vi "Connection Engine.vi"(8 "error in (no error)":errorcluster, 11 "State Variables":T1={"TCP Refs"={"Connection List"=refnum, "listener ID"=refnum}, "Stop"=refnum, "Top VI"=refnum, "Parameters"={"Properties"={"Name"="", "CAN"={"Database File"=path "", "CAN Interface"=enum."CAN0", "Baud Rate"=0, "Diagnostic Protocol"=enum."GMLAN", "Transport Protocol"=enum."ISO TP - Normal Mode", "Transmit ID"=0, "Receive ID"=0, "Transmit Extension"=0, "Receive Extension"=0, "Receive UUDT ID"=0, "Enable Stream"=TRUE, "VW TP Channel ID"=0, "Security"={"DLL Path"=path "", "Security Level"=1}}, "FPGA Settings"={"RT Bitfile Path"=path "", "RIO Device"=0, "Enable"=FALSE}, "PIDs"=[], "PID Lookup"=variant, "CPIDs"=[], "CPID Lookup"=variant, "DIDs"=[], "DID Lookup"=variant, "DPIDs"=[], "DPID Lookup"=variant, "DTC descriptor"={"DTC Byte Length"=2, "Status Byte Length"=1, "Add Data Byte Length"=1, "Byte Order"=enum."Motorola"}}, "ChanRefs"={"ToVS.PIDs"={"Name"="", "Write to VS Engine FIFO"=refnum, "Pairs"={"Refs"=[], "Values"=[]}}, "ToVS.DIDs"={"Name"="", "Write to VS Engine FIFO"=refnum, "Pairs"={"Refs"=[], "Values"=[]}}, "ToVS.DTCs"={"Name"="", "Write to VS Engine FIFO"=refnum, "Pairs"={"Refs"=[], "Values"=[]}}, "ToVS.DTCCount"={"Name"="", "Write to VS Engine FIFO"=refnum, "Pairs"={"Refs"=[], "Values"=[]}}, "ToVS.Success"={"Name"="", "Write to VS Engine FIFO"=refnum, "Pairs"={"Refs"=[], "Values"=[]}}, "FromVS.CPIDs"={"Name"="", "Read from VS Engine FIFO"=refnum, "Pairs"={"Refs"=[], "Values"=[]}}, "Cmds"={"Name"="", "Write to VS Engine FIFO"=refnum, "Read from VS Engine FIFO"=refnum, "Pairs"={"Chan Refs"=[], "Prev. Values"=[]}}}}, "ADCS Connection"={"Diag CAN Handle"=0, "Transport Protocol"=enum."ISO TP - Normal Mode", "Receive Address Extension"=0, "Transmit Address Extension"=0, "Receive CAN Id"=0, "Transmit CAN Id"=0, "Diag CAN Queue"=refnum, "Log Frames ?"=FALSE, "My TP Address"=0, "Other TP Address"=0, "T1"=0, "T2"=0, "T3"=0, "T4"=0, "Tx SN"=0, "Block Size"=0, "Rx SN"=0, "VW TP Initialized?"=FALSE, "Tx block no"=0, "baud rate"=0, "Interface"="", "Channel Diag CAN Handle"=0, "UDP Connection ID"=refnum, "TCP Connection ID"=refnum, "Target IP Addr"=0, "Source Address"=0, "Target Address"=0, "Send Header NACK?"=FALSE, "DLL Handle"=0, "NAD"=0, "Time Stamp read first"=0.0, "Time Stamp read last"=0.0, "Time Stamp write first"=0.0, "Time Stamp write last"=0.0, "Time Stamp write"=0.0, "Time Stamp read"=0.0}, "XNET References"={"Database"="", "GMLAN DPID Session"="", "Cluster"=""}, "BufferedCmds"=refnum, "XNETEngine (GMLAN)"=refnum} {"Parameters"."ChanRefs"."Cmds"."Pairs"."Chan Refs" format="%.0x"; "Parameters"."ChanRefs"."ToVS.Success"."Pairs"."Refs" format="%.0x"; "Parameters"."ChanRefs"."ToVS.DTCCount"."Pairs"."Refs" format="%.0x"; "Parameters"."ChanRefs"."ToVS.DTCs"."Pairs"."Refs" format="%.0x"; "Parameters"."ChanRefs"."ToVS.PIDs"."Pairs"."Refs" format="%.0x"; "Parameters"."ChanRefs"."ToVS.DIDs"."Pairs"."Refs" format="%.0x"; "Parameters"."Properties"."CPIDs"."Signals"."Byte Order" items=["Little Endian", "Big Endian"]; "Parameters"."Properties"."CPIDs"."Signals"."Data Type" items=["Signed", "Unsigned", "IEEE Float"]; "Parameters"."Properties"."DIDs"."Signals"."Byte Order" items=["Little Endian", "Big Endian"]; "Parameters"."Properties"."DIDs"."Signals"."Data Type" items=["Signed", "Unsigned", "IEEE Float"]; "Parameters"."Properties"."CAN"."VW TP Channel ID" format="%.0x"; "Parameters"."Properties"."CAN"."Receive UUDT ID" format="%.0x"; "Parameters"."Properties"."CAN"."Receive Extension" format="%.0x"; "Parameters"."Properties"."CAN"."Transmit Extension" format="%.0x"; "Parameters"."Properties"."CAN"."Receive ID" format="%.0x"; "Parameters"."Properties"."CAN"."Transmit ID" format="%.0x"; "Parameters"."Properties"."PIDs"."Signals"."Byte Order" items=["Little Endian", "Big Endian"]; "Parameters"."Properties"."PIDs"."Signals"."Data Type" items=["Signed", "Unsigned", "IEEE Float"]}) -> (0 "error out":errorcluster)   [LabVIEW 2015, in "Diagnostics Addon Engine.lvlib"]
uses:
  Diagnostics Addon Engine.lvlib
  Stop FG/Stop Global Commands.ctl
  Stop FG/Stop FG.lvlib
  STM/TCP/stm_TCP Read Options.ctl
  STM/Connection Manager/stm_TCPConnectionMethod.ctl
  STM/Connection Manager/stm_TCPConnectionProperties.ctl
  <vilib>/NI Veristand/Custom Device Tools/Custom Device Utility Library/Custom Device Utility Library.lvlib
  STM/TCP/STM Read Meta Data (TCP Ref).vi
  Error Handling API/Error Handling API.lvlib
  STM/STM Lookup Table Ref.ctl
  TCP Refs.ctl
  State Variables.ctl
  Shared/Diagnostic Protocols.ctl
  Shared/Diagnostics Addon Shared.lvlib
  Shared/CAN Interface.ctl
  Shared/CAN Configuration.ctl
  <vilib>/Automotive Diagnostic Command Set/Diagnostic Protocols.llb/DTC Descriptor.ctl
  Main Configuration.ctl
  Shared/Signal Parameters.ctl
  Shared/Frame Parameters.ctl
  Shared/DPID Periodic Rate.ctl
  Shared/DPID Parameters.ctl
  Section Properties.ctl
  XNET References.ctl
  <vilib>/NI Veristand/Custom Device API/Data Reference.ctl
  <vilib>/NI Veristand/Custom Device API/Custom Device API.lvlib
  VS Data Channels.ctl
  <vilib>/NI Veristand/Custom Device API/Block Data Reference.ctl
  <vilib>/NI/Tools/Keyed Array/KeyedArray.ctl
  <vilib>/NI/Tools/Keyed Array/Tools_KeyedArray.lvlib
  <vilib>/NI/AMC/Message.ctl
  <vilib>/NI/AMC/AMC.lvlib
  <vilib>/NI/AMC/Message Queue.ctl
  Shared/Transport Protocols.ctl
  <vilib>/Automotive Diagnostic Command Set/Diagnostic Transport.llb/Transport Protocol Selector.ctl
  <vilib>/addons/Automotive Diagnostic Command Set/NI_Automotive Diagnostic Command Set.lvlib
  <vilib>/Automotive Diagnostic Command Set/Diagnostic Transport.llb/Diag CAN Frame Log.ctl
  <vilib>/Automotive Diagnostic Command Set/Diagnostic Transport.llb/Diag Reference.ctl
  Inline Async API/Controls/Write To VS Engine.ctl
  Inline Async API/Inline Async API.lvlib
  Inline Async API/Controls/Read From VS Engine.ctl
  Inline Async API/Controls/ReadWrite Data.ctl
  Stop FG/Stop Global Ref.ctl
  Shared/Security.ctl
  Shared/FPGA Bitfile Settings.ctl
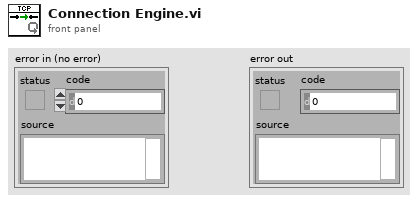
[diagram p1: front panel]
types:
  T1 = typedef "Diagnostics Addon Engine.lvlib/State Variables.ctl" = cluster{"TCP Refs":T2, "Stop":T4, "Top VI":refnum<vi>, "Parameters":T5, "ADCS Connection":T24, "XNET References":T26, "BufferedCmds":T27, "XNETEngine (GMLAN)":T27}
  T2 = typedef "Diagnostics Addon Engine.lvlib/TCP Refs.ctl" = cluster{"Connection List":T3, "listener ID":refnum<k5>}
  T3 = typedef "Diagnostics Addon Engine.lvlib/STM Lookup Table Ref.ctl" = refnum<vi>
  T4 = typedef "Diagnostics Addon Engine.lvlib/Stop FG.lvlib/Stop Global Ref.ctl" = refnum<vi>
  T5 = typedef "Diagnostics Addon Engine.lvlib/Main Configuration.ctl" = cluster{"Properties":T6, "ChanRefs":T18}
  T6 = typedef "Diagnostics Addon Engine.lvlib/Section Properties.ctl" = cluster{"Name":string, "CAN":T7, "FPGA Settings":T12, "PIDs":T13[], "PID Lookup":variant, "CPIDs":T13[], "CPID Lookup":variant, "DIDs":T13[], "DID Lookup":variant, "DPIDs":T15[], "DPID Lookup":variant, "DTC descriptor":T17}
  T7 = typedef "Diagnostics Addon Shared.lvlib/CAN Configuration.ctl" = cluster{"Database File":path, "CAN Interface":T8, "Baud Rate":u32, "Diagnostic Protocol":T9, "Transport Protocol":T10, "Transmit ID":u32, "Receive ID":u32, "Transmit Extension":u8, "Receive Extension":u8, "Receive UUDT ID":u32, "Enable Stream":bool, "VW TP Channel ID":u32, "Security":T11}
  T8 = typedef "Diagnostics Addon Shared.lvlib/CAN Interface.ctl" = enum16{"CAN0", "CAN1", "CAN2", "CAN3", "CAN4", "CAN5", "CAN6", "CAN7", "CAN8", "CAN9", "CAN10", "CAN11", "CAN12", "CAN13", "CAN14", "CAN15", "CAN16", "CAN17", "CAN18", "CAN19", "CAN20", "CAN21", "CAN22", "CAN23", "CAN24", "CAN25", "CAN26", "CAN27", "CAN28", "CAN29", "CAN30", "CAN31", "CAN32", "CAN33", "CAN34", "CAN35", "CAN36", "CAN37", "CAN38", "CAN39", "CAN40", "CAN41", "CAN42", "CAN43", "CAN44", "CAN45", "CAN46", "CAN47", "CAN48", "CAN49", "CAN50", "CAN51", "CAN52", "CAN53", "CAN54", "CAN55", "CAN56", "CAN57", "CAN58", "CAN59", "CAN60", "CAN61", "CAN62", "CAN63", "CAN 256 (Virtual)", "CAN 257 (Virtual)"}
  T9 = typedef "Diagnostics Addon Shared.lvlib/Diagnostic Protocols.ctl" = enum16{"GMLAN", "KWP-2000", "UDS"}
  T10 = typedef "Diagnostics Addon Shared.lvlib/Transport Protocols.ctl" = enum16{"ISO TP - Normal Mode", "ISO TP - Mixed Mode", "VW TP 2.0", "Diagnostics on IP"}
  T11 = typedef "Diagnostics Addon Shared.lvlib/Security.ctl" = cluster{"DLL Path":path, "Security Level":u8}
  T12 = typedef "Diagnostics Addon Shared.lvlib/FPGA Bitfile Settings.ctl" = cluster{"RT Bitfile Path":path, "RIO Device":u16, "Enable":bool}
  T13 = typedef "Diagnostics Addon Shared.lvlib/Frame Parameters.ctl" = cluster{"Name":string, "Description":string, "ID":u16, "Signals":T14[]}
  T14 = typedef "Diagnostics Addon Shared.lvlib/Signal Parameters.ctl" = cluster{"Start Bit":u8, "Length":u8, "Scaling Factor":dbl, "Scaling Offset":dbl, "Minimum":dbl, "Maximum":dbl, "Data Type":u32, "Byte Order":u32, "Default Value":dbl, "Name":string, "Units":string, "Description":string}
  T15 = typedef "Diagnostics Addon Shared.lvlib/DPID Parameters.ctl" = cluster{"DPID ID":u8, "Speed":T16, "PIDs":u16[]}
  T16 = typedef "Diagnostics Addon Shared.lvlib/DPID Periodic Rate.ctl" = enum16{"Slow", "Medium", "Fast"}
  T17 = typedef "Diagnostics Addon Shared.lvlib/DTC Descriptor.ctl" = cluster{"DTC Byte Length":i32, "Status Byte Length":i32, "Add Data Byte Length":i32, "Byte Order":enum16{"Motorola", "Intel"}}
  T18 = typedef "Diagnostics Addon Engine.lvlib/VS Data Channels.ctl" = cluster{"ToVS.PIDs":T19, "ToVS.DIDs":T19, "ToVS.DTCs":T19, "ToVS.DTCCount":T19, "ToVS.Success":T19, "FromVS.CPIDs":T21, "Cmds":T23}
  T19 = typedef "Diagnostics Addon Engine.lvlib/Inline Async API.lvlib/Write To VS Engine.ctl" = cluster{"Name":string, "Write to VS Engine FIFO":refnum<k33>, "Pairs":cluster{"Refs":T20[], "Values":dbl[]}}
  T20 = typedef "Custom Device API.lvlib/Data Reference.ctl" = i32
  T21 = typedef "Diagnostics Addon Engine.lvlib/Inline Async API.lvlib/Read From VS Engine.ctl" = cluster{"Name":string, "Read from VS Engine FIFO":refnum<k33>, "Pairs":cluster{"Refs":T22[], "Values":dbl[]}}
  T22 = typedef "Custom Device API.lvlib/Block Data Reference.ctl" = cluster{"Data Reference":T20, "Offset":u64, "Length":u64}
  T23 = typedef "Diagnostics Addon Engine.lvlib/Inline Async API.lvlib/ReadWrite Data.ctl" = cluster{"Name":string, "Write to VS Engine FIFO":refnum<k33>, "Read from VS Engine FIFO":refnum<k33>, "Pairs":cluster{"Chan Refs":T20[], "Prev. Values":dbl[]}}
  T24 = typedef "NI_Automotive Diagnostic Command Set.lvlib/Diag Reference.ctl" = cluster{"Diag CAN Handle":u32, "Transport Protocol":T25, "Receive Address Extension":u8, "Transmit Address Extension":u8, "Receive CAN Id":u32, "Transmit CAN Id":u32, "Diag CAN Queue":refnum<queue>, "Log Frames ?":bool, "My TP Address":u8, "Other TP Address":u8, "T1":u16, "T2":u16, "T3":u16, "T4":u16, "Tx SN":u8, "Block Size":u8, "Rx SN":u8, "VW TP Initialized?":bool, "Tx block no":u8, "baud rate":u32, "Interface":string, "Channel Diag CAN Handle":u32, "UDP Connection ID":refnum<k16>, "TCP Connection ID":refnum<k5>, "Target IP Addr":u32, "Source Address":u16, "Target Address":u16, "Send Header NACK?":bool, "DLL Handle":u32, "NAD":u8, "Time Stamp read first":dbl, "Time Stamp read last":dbl, "Time Stamp write first":dbl, "Time Stamp write last":dbl, "Time Stamp write":dbl, "Time Stamp read":dbl}
  T25 = typedef "NI_Automotive Diagnostic Command Set.lvlib/Transport Protocol Selector.ctl" = enum16{"ISO TP - Normal Mode", "ISO TP - Mixed Mode", "VW TP 2.0", "Diagnostics on IP", "ISO TP LIN"}
  T26 = typedef "Diagnostics Addon Engine.lvlib/XNET References.ctl" = cluster{"Database":refnum<k21>, "GMLAN DPID Session":refnum<k21>, "Cluster":refnum<k21>}
  T27 = typedef "AMC.lvlib/Message Queue.ctl" = refnum<queue>
  T28 = typedef "Diagnostics Addon Engine.lvlib/Stop FG.lvlib/Stop Global Commands.ctl" = enum16{"Write", "Read", "Reset"}
  T29 = typedef "Diagnostics Addon Engine.lvlib/stm_TCP Read Options.ctl" = cluster{"Ignore Timeout Error":bool, "timeout ms (1000)":i32}
  T30 = typedef "Diagnostics Addon Engine.lvlib/stm_TCPConnectionProperties.ctl" = cluster{"Name":string, "Address":string, "Custom":string}
  T31 = typedef "Diagnostics Addon Engine.lvlib/stm_TCPConnectionMethod.ctl" = enum16{"Initialize", "Add Connection", "Set Properties", "Get Connection(s)", "Remove Connection", "Remove All Connections", "Get Connection Count"}
  T32 = typedef "Diagnostics Addon Engine.lvlib/stm_TCP Connection Info.ctl" = cluster{"connection ID":refnum<k5>, "Meta data":T33[]}
  T33 = typedef "Diagnostics Addon Engine.lvlib/stm_MetaDataElement.ctl" = string
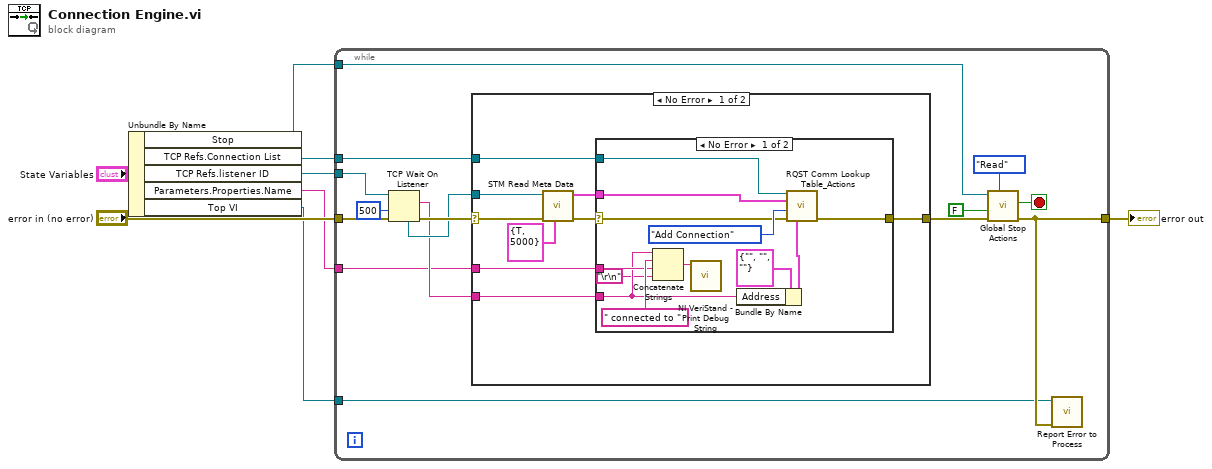
[diagram p0: block diagram]
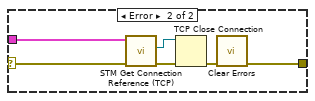
[diagram p2: hidden frame]
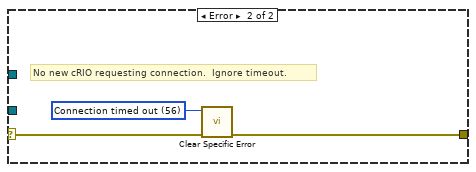
[diagram p3: hidden frame]
diagram:
  n1 = Unbundle By Name("State Variables") -> ("Stop"=w8:T4, "TCP Refs.Connection List"=w6:T3, "TCP Refs.listener ID"=w7:refnum<k5>, "Parameters.Properties.Name"=w1:string, "Top VI"=w2:refnum<vi>)
  n2 = while {
    tunnel: "error in (no error)" -> [w23]
    tunnel: w7 -> [w22]
    tunnel: w8 -> [w15]
    tunnel: [w12] -> w3
    tunnel: w6 -> [w13]
    tunnel: w1 -> [w11]
    tunnel: w2 -> [w9]
    stop <- w17 stop-if-true
    n3 = TCP Wait On Listener(8:w23, 9:500 ("timeout ms (wait forever: -1)"), 11:w22) -> (0:w20:errorcluster, 2:w18:string, 4:w19:refnum<k5>)  [unwired: 1 in, 2 out]
    n4 = case shown="No Error" w20 {
      selector: w20 -> [w32 w53]
      tunnel: w19 -> [w26 _]
      tunnel: [w30 w52] -> w16
      tunnel: w18 -> [w28 _]
      tunnel: w13 -> [w29 _]
      tunnel: w11 -> [w27 _]
      frame No Error {
        n5 = call-poly "STM Read Meta Data.vi"("Options"=T29 {"Ignore Timeout Error"=TRUE, "timeout ms (1000)"=5000}, "error in"=w32, "connection ID"=w26) -> ("error out"=w25:errorcluster, "Connection Info Out"=w24:T32)  [unwired: 6 in, 1 out]
        n6 = case shown="No Error" w25 {
          selector: w25 -> [w40 w49]
          tunnel: w29 -> [w38 _]
          tunnel: w24 -> [w39 w48]
          tunnel: [w41 w50] -> w30
          tunnel: w28 -> [w34 _]
          tunnel: w27 -> [w35 _]
          frame No Error {
            n7 = Concatenate Strings(w34, " connected to " ("string"), w35, "\r\n") -> (w36:string)
            n8 = call <vilib>:"NI VeriStand - Print Debug String.vi"("Message"=w36) -> ()  [unwired: 10 in, 1 out]
            n9 = Bundle By Name(cluster=T30 {"Name"="", "Address"="", "Custom"=""} ("Properties In"), "Address"=w34) -> (w44:T30)
            n10 = call "RQST Comm Lookup Table_Actions.vi"("ref in"=w38, "Connection In"=w39, "Method"=stm_TCPConnectionMethod."Add Connection", "error in (no error)"=w40, "Properties In"=w44) -> ("error out"=w41:errorcluster)  [unwired: 4 in, 6 out]
          }
          frame Error {
            n11 = call "STM Get Connection Reference (TCP).vi"("error in"=w49, "Connection Info"=w48) -> ("error out"=w47:errorcluster, "connection ID out"=w46:refnum<k5>)  [unwired: 7 in, 1 out]
            n12 = TCP Close Connection(connection ID=w46, error in (no error)=w47) -> (error out=w45:errorcluster)  [unwired: 1 in, 1 out]
            n13 = call <vilib>:"Clear Errors.vi"("error in (no error)"=w45) -> ("error out"=w50:errorcluster)  [unwired: 5 in, 1 out]
          }
        }
      }
      frame Error {
        w51 = 56 items=["No Error", "Argument Error", "Memory Full", "Out of Zone", "End of File", "File Already Open", "Generic File IO Error", "File Not Found", "File Permission Error", "Disk Full", "Duplicate Path", "Too Many Files Open", "Not Enabled", "Resource File Not Found", "Cannot Add Resource", "Resource Not Found", "Image Not Found", "Image Memory Error", "Pen Does Not Exist", "Config Bad Type", "Config Token Not Found", "Config Parse Error", "Config Memory Error", "Bad External Code Format", "Bad External Code Offset", "External Code Not Present", "Null Window", "Destroy Window Mixup", "Null Menu", "Print Aborted", "Bad Print Record", "Print Driver Error", "Windows Error During Print", "Memory Error During Print", "Print Dialog Error", "Generic Print Error", "Invalid Device Refnum", "Device Not Found", "Device Parameter Error", "Device Unit Error", "Can't Open Device", "Device Call Aborted", "Generic Error", "Cancelled By User", "Object ID Too Low", "Object ID Too High", "Object Not In Heap", "Unknown Heap", "Bad DefProc ID", "DefProc Not In Table", "Message Out Of Range", "Null Method", "Unknown Message", "Manager Call Not Supported", "Bad address", "Connection In progress", "Connection timed out", "Connection is already in progress", "Network attribute not supported", "Network error", "Address in use", "System out of memory", "Connection aborted", "Connection refused", "Connection is not connected", "Connection is already connected", "Connection closed", "Initialize error (interapplication manager)", "Bad occurrence", "Wait on unbound occurrence handler", "Occurrence queue overflow", "Bad path", "Semaphore not signaled", "Unrecognized type (interapplication manager)"] ("1st Error to Convert")
        # "No new cRIO requesting connection.  Ignore timeout."
        n14 = call "Clear Specific Error.vi"("error in (no error)"=w53, "code"=w51) -> ("error out"=w52:errorcluster)  [unwired: 9 out]
      }
    }
    n15 = call "Global Stop Actions.vi"("Command"=Stop_Global_Commands."Read", "error in (no error)"=w16, "Stop on Error?"=FALSE, "vi reference"=w15) -> ("error out"=w12:errorcluster, "Latched Stop"=w17:bool)  [unwired: 5 in, 1 out]
    n16 = call "Report Error to Process.vi"("Error"=w12, "This VI"=w9) -> ()  [unwired: 10 in]
  }
  "error out" <- w3
